vi "Read Application Style Reference.vi"(11 "IViewable in":refnum<class "IViewable.lvclass">) -> (2 "Application Style Reference":T1)   [LabVIEW 2018, in "MVA Framework.lvlib" / "IViewable.lvlib" / "IViewable.lvclass"]
doc: "读取应用程序样式引用"
uses:
  IViewable.lvclass
  ApplicationStyleReference/ApplicationStyleReference.lvclass
  ApplicationStyleReference/Application Style Reference.ctl
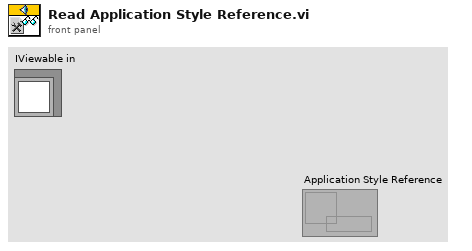
[diagram p1: front panel]
types:
  T1 = typedef "MVA Framework.lvlib/IViewable.lvlib/ApplicationStyleReference.lvclass/Application Style Reference.ctl" = refnum<data-value>
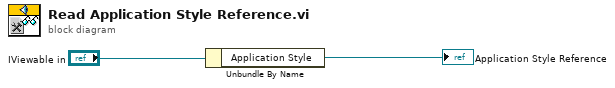
[diagram p0: block diagram]
diagram:
  n1 = Unbundle By Name("IViewable in") -> ("Application Style"=→"Application Style Reference":T1)
